vi "getTaskReference.vi"(8 "error in (no error)":errorcluster, 11 "ExampleTask_MsgUserEventStopNotifier In":refnum<class "Task_MsgUserEventStopMech.lvclass">) -> (0 "error out":errorcluster, 2 "taskRef":refnum<vi>, 3 "ExampleTask_MsgUserEventStopNotifier Out":refnum<class "Task_MsgUserEventStopMech.lvclass">)   [LabVIEW 2023, in "Task_MsgUserEventStopMech.lvclass"]
doc: "Returns the VI reference related to the task to handle."
uses:
  Task_MsgUserEventStopMech.lvclass
  myTask.vi
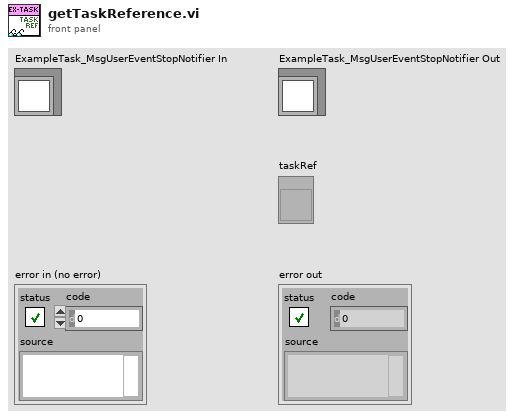
[diagram p1: front panel]
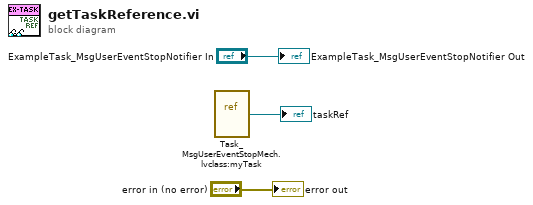
[diagram p0: block diagram]
diagram:
  n1 = vi-ref "Task_MsgUserEventStopMech.lvclass:myTask.vi"() -> (→"taskRef":refnum<vi>)
  "error out" <- "error in (no error)"
  "ExampleTask_MsgUserEventStopNotifier Out" <- "ExampleTask_MsgUserEventStopNotifier In"
